vi "Test Summary Page.vi"(8 "error in (no error)":errorcluster, 9 "GC Config":T3, 10 "Test Results":T1, 11 "Type":string="Step") -> (0 "error out":errorcluster, 3 "Result":bool)   [LabVIEW 2015]
uses:
  Tests/Controls/Test Information.ctl
  Tests/Controls/Vacuum Test.ctl
  Tests/Controls/Test Timing.ctl
  Tests/Controls/Vaccum Thresholds.ctl
  Tests/Controls/Helium Test.ctl
  Tests/Controls/Helium Thresholds.ctl
  Tests/Controls/Test Results.ctl
  Tests/Controls/Step Result.ctl
panel:
  out "String Result":string
  in  "OK":bool
  in  "Thresholds":i32(listbox)=-1
  # "Test Result Summary"
  # "Result"
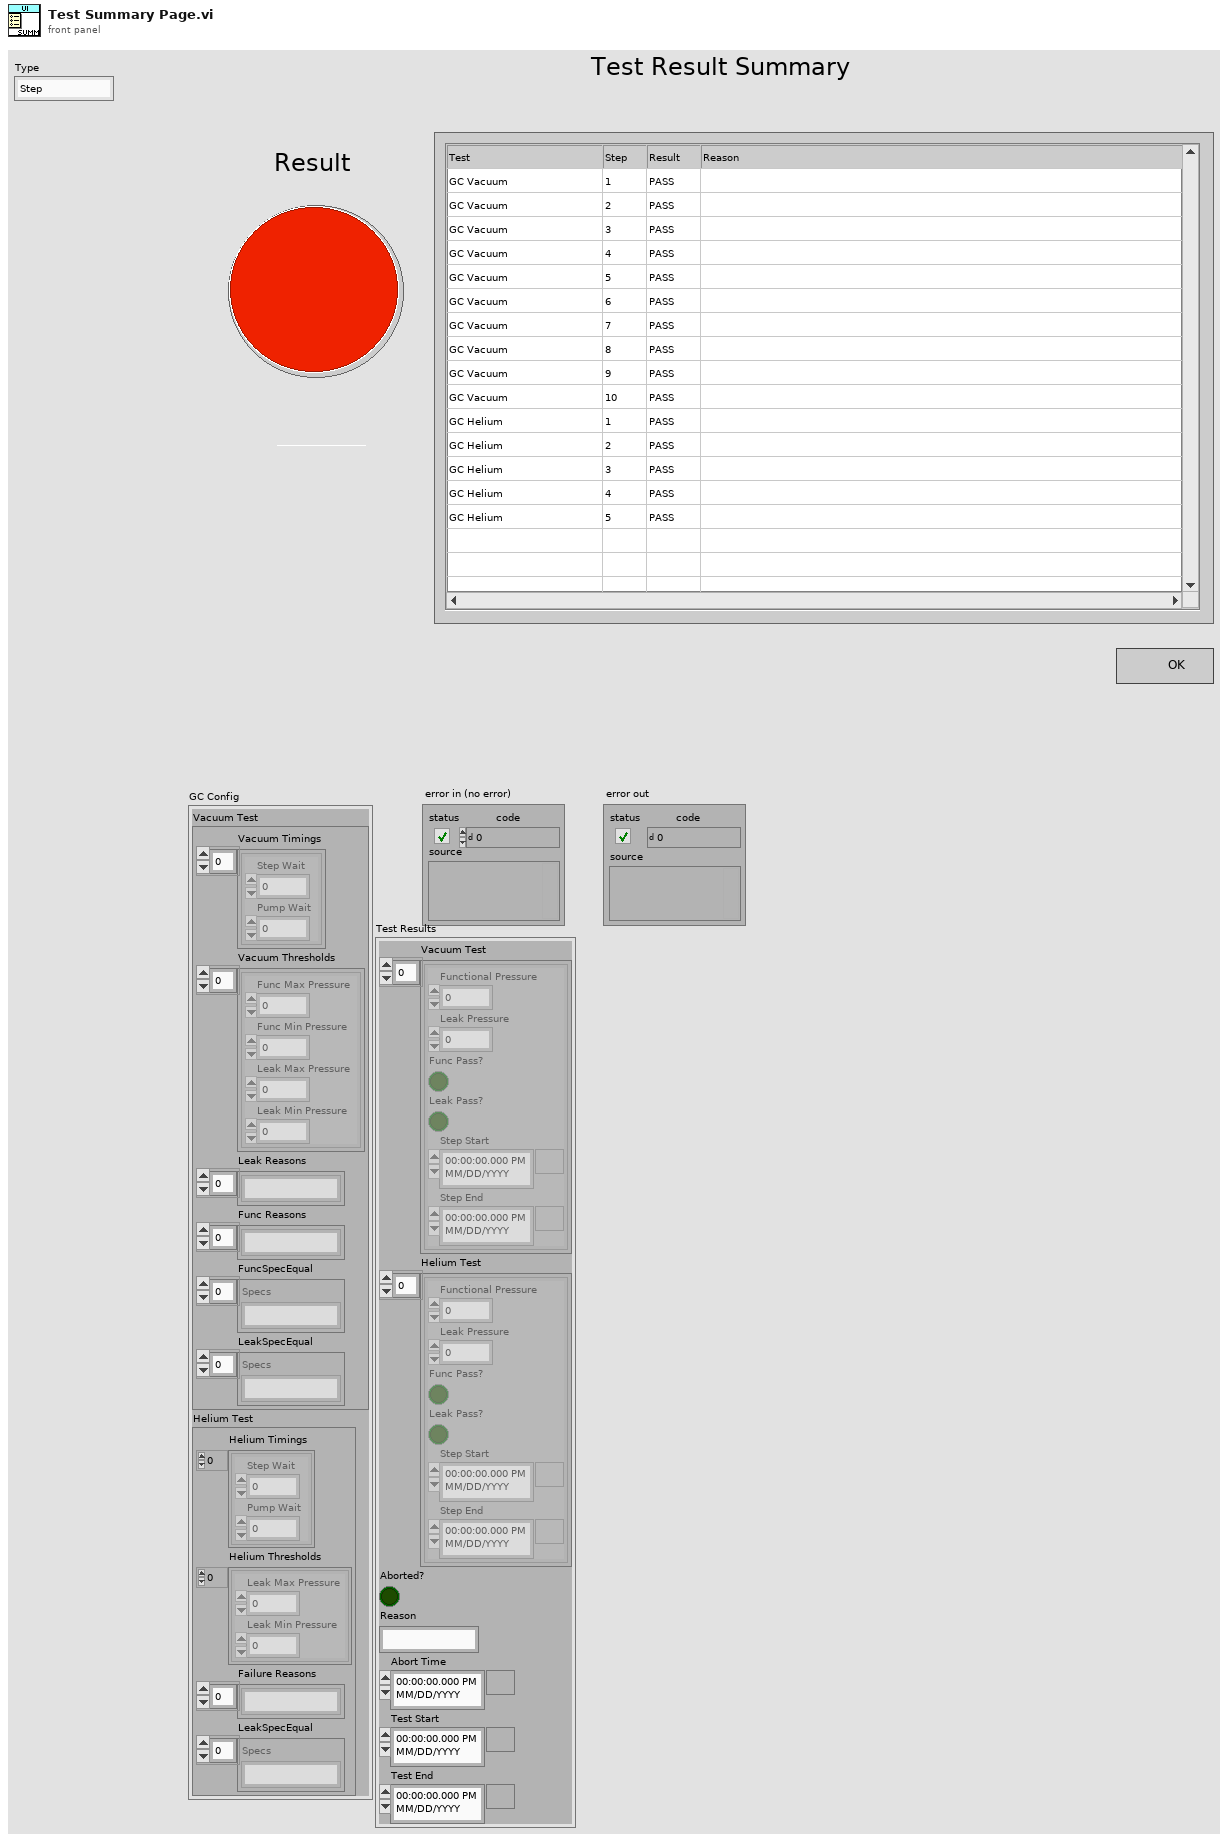
[diagram p1: front panel]
types:
  T1 = typedef "Test Results.ctl" = cluster{"Vacuum Test":T2[], "Helium Test":T2[], "Aborted?":bool, "Reason":string, "Abort Time":timestamp, "Test Start":timestamp, "Test End":timestamp}
  T2 = typedef "Step Result.ctl" = cluster{"Functional Pressure":dbl, "Leak Pressure":dbl, "Func Pass?":bool, "Leak Pass?":bool, "Step Start":timestamp, "Step End":timestamp}
  T3 = typedef "Test Information.ctl" = cluster{"Vacuum Test":T4, "Helium Test":T7}
  T4 = typedef "Vacuum Test.ctl" = cluster{"Vacuum Timings":T5[], "Vacuum Thresholds":T6[], "Leak Reasons":string[], "Func Reasons":string[], "FuncSpecEqual":string[], "LeakSpecEqual":string[]}
  T5 = typedef "Test Timing.ctl" = cluster{"Step Wait":dbl, "Pump Wait":dbl}
  T6 = typedef "Vaccum Thresholds.ctl" = cluster{"Func Max Pressure":dbl, "Func Min Pressure":dbl, "Leak Max Pressure":dbl, "Leak Min Pressure":dbl}
  T7 = typedef "Helium Test.ctl" = cluster{"Helium Timings":T5[], "Helium Thresholds":T8[], "Failure Reasons":string[], "LeakSpecEqual":string[]}
  T8 = typedef "Helium Thresholds.ctl" = cluster{"Leak Max Pressure":dbl, "Leak Min Pressure":dbl}
  T9 = typedef "LVPoint32TypeDef.ctl" = cluster{"Horizontal":i32, "Vertical":i32}
  T10 = typedef "LVRowAndColumnTypeDef.ctl" = cluster{"Row":i32, "Column":i32}
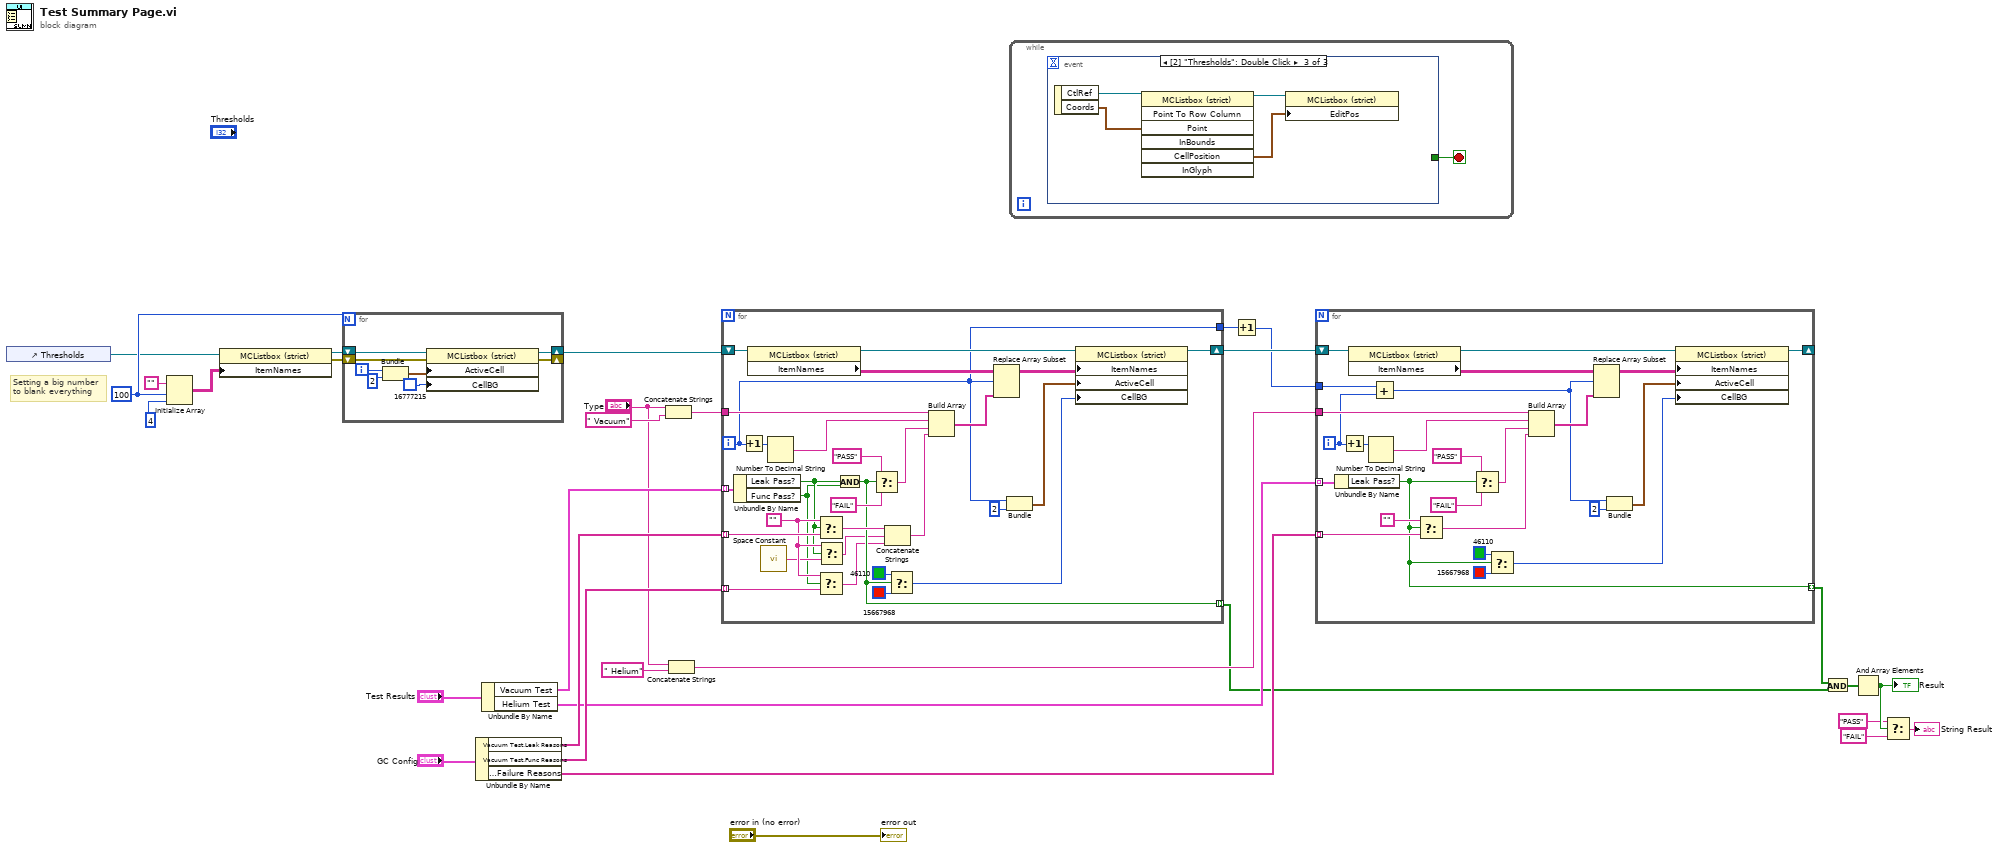
[diagram p0: block diagram]
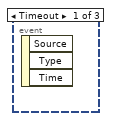
[diagram p2: hidden frame]
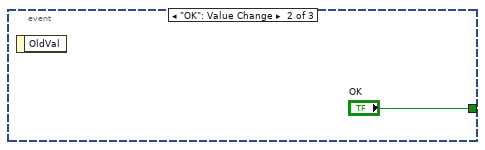
[diagram p3: hidden frame]
diagram:
  w11 = 100 ("dimension size")
  # "Setting a big number\nto blank everything"
  n1 = control-ref of="Thresholds"() -> (w10:refnum<vi>)
  n2 = Initialize Array("", w11, 4 ("dimension size")) -> (w15:string[][])
  n3 = property class="MCListbox (strict)"(reference=w10, "ItemNames"=w15) -> (reference out=w14:refnum<vi>, error out=w13:errorcluster)  [unwired: 1 in]
  n4 = for {
    N: w11 -> [_]
    shift-right: [w38] -> w9
    shift-left: w14 -> [w39]
    shift-right: [w32] -> _
    shift-left: w13 -> [w33]
    i -> [w37]
    n5 = Bundle(w37, "element"=2) -> (w35:cluster{i32, "element":i32})  [unwired: 1 in]
    n6 = property class="MCListbox (strict)"(reference=w39, error in=w33, "ActiveCell"=w35, "CellBG"=u32 16777215) -> (reference out=w38:refnum<vi>, error out=w32:errorcluster)
  }
  n7 = Unbundle By Name("GC Config") -> ("Vacuum Test.Leak Reasons"=w27:string[], "Vacuum Test.Func Reasons"=w26:string[], "Helium Test.Failure Reasons"=w21:string[])
  n8 = Unbundle By Name("Test Results") -> ("Vacuum Test"=w31:T2[], "Helium Test"=w22:T2[])
  n9 = Concatenate Strings("Type", " Vacuum") -> (w29:string)
  n10 = Concatenate Strings("Type", " Helium") -> (w23:string)
  n11 = for {
    tunnel: w31 -> [w69] mode=indexing
    tunnel: w29 -> [w65]
    tunnel: w27 -> [w62] mode=indexing
    tunnel: w26 -> [w61] mode=indexing
    shift-right: [w53] -> w25
    shift-left: w9 -> [w58]
    tunnel: [w47] -> w8 mode=indexing
    tunnel: [w46] -> w20
    i -> [w46]
    w44 = ""
    n12 = Unbundle By Name(w69) -> ("Leak Pass?"=w41:bool, "Func Pass?"=w40:bool)
    n13 = Increment(x=w46) -> (x+1=w68:i32)
    n14 = property class="MCListbox (strict)"(reference=w58) -> (reference out=w55:refnum<vi>, "ItemNames"=w57:string[][])  [unwired: 1 in, 1 out]
    n15 = call <vilib>:"Space Constant.vi"() -> ("String"=w43:string)
    n16 = Number To Decimal String(number=w68) -> (decimal integer string=w64:string)  [unwired: 1 in]
    n17 = Select(t=w44, s=w41, f=w62) -> (s? t:f=w60:string)
    n18 = Select(t=w44, s=w40, f=w61) -> (s? t:f=w45:string)
    n19 = Select(t=w44, s=w41, f=w43) -> (s? t:f=w42:string)
    n20 = And(x=w41, y=w40) -> (x .and. y?=w47:bool)
    n21 = Select(t="PASS", s=w47, f="FAIL") -> (s? t:f=w63:string)
    n22 = Concatenate Strings(w60, w42, w45) -> (w59:string)
    n23 = Select(t=u32 46110, s=w47, f=u32 15667968) -> (s? t:f=w48:u32)
    n24 = Build Array(w65, w64, w63, w59) -> (w56:string[])
    n25 = Replace Array Subset(array=w57, new element=w56, index (row)=w46) -> (w54:string[][])  [unwired: 1 in]
    n26 = Bundle(w46, 2) -> (w51:cluster{i32, i32})  [unwired: 1 in]
    n27 = property class="MCListbox (strict)"(reference=w55, "ItemNames"=w54, "ActiveCell"=w51, "CellBG"=w48) -> (reference out=w53:refnum<vi>)  [unwired: 1 in, 1 out]
  }
  n28 = while {
    stop <- w70 stop-if-true
    n29 = event shown="[2] \"Thresholds\": Double Click" {
      selector: _ -> [_ _ _]
      dyn-events: _ -> [_ _ _]
      timeout: _ -> [_ _ _]
      tunnel: [_ "OK" _] -> w70
      event Timeout {
        n30 = event-data() -> ()  [unwired: 1 in, 3 out]
      }
      event "OK": Value Change {
        n31 = event-data() -> ()  [unwired: 1 in, 1 out]
      }
      event "Thresholds": Double Click {
        n32 = event-data() -> ("CtlRef"=w75:refnum<vi>, "Coords"=w74:T9)  [unwired: 1 in]
        n33 = invoke class="MCListbox (strict)" method="Point To Row Column"(reference=w75, "Point"=w74) -> (reference out=w73:refnum<vi>, "CellPosition"=w72:T10)  [unwired: 5 in, 5 out]
        n34 = property class="MCListbox (strict)"(reference=w73, "EditPos"=w72) -> ()  [unwired: 1 in, 2 out]
      }
    }
  }
  n35 = Increment(x=w20) -> (x+1=w19:i32)
  n36 = for {
    tunnel: w22 -> [w100] mode=indexing
    tunnel: w23 -> [w96]
    tunnel: w21 -> [w93] mode=indexing
    shift-right: [w87] -> _
    shift-left: w25 -> [w92]
    tunnel: w19 -> [w79]
    tunnel: [w76] -> w1 mode=indexing
    i -> [w78]
    n37 = Unbundle By Name(w100) -> ("Leak Pass?"=w76:bool)
    n38 = Increment(x=w78) -> (x+1=w99:i32)
    n39 = property class="MCListbox (strict)"(reference=w92) -> (reference out=w89:refnum<vi>, "ItemNames"=w91:string[][])  [unwired: 1 in, 1 out]
    n40 = Number To Decimal String(number=w99) -> (decimal integer string=w95:string)  [unwired: 1 in]
    n41 = Add(x=w79, y=w78) -> (x+y=w77:i32)
    n42 = Select(t="", s=w76, f=w93) -> (s? t:f=w80:string)
    n43 = Select(t="PASS", s=w76, f="FAIL") -> (s? t:f=w94:string)
    n44 = Select(t=u32 46110, s=w76, f=u32 15667968) -> (s? t:f=w82:u32)
    n45 = Build Array(w96, w95, w94, w80) -> (w90:string[])
    n46 = Replace Array Subset(array=w91, new element=w90, index (row)=w77) -> (w88:string[][])  [unwired: 1 in]
    n47 = Bundle(w77, 2) -> (w85:cluster{i32, i32})  [unwired: 1 in]
    n48 = property class="MCListbox (strict)"(reference=w89, "ItemNames"=w88, "ActiveCell"=w85, "CellBG"=w82) -> (reference out=w87:refnum<vi>)  [unwired: 1 in, 1 out]
  }
  n49 = And(x=w1, y=w8) -> (x .and. y?=w18:bool[])
  n50 = And Array Elements(Boolean array=w18) -> (logical AND=w7:bool)
  "Result" <- w7
  n51 = Select(t="PASS", s=w7, f="FAIL") -> (s? t:f=→"String Result":string)
  "error out" <- "error in (no error)"
